vi "Launch Quad With Play and Pause.vi"   [LabVIEW 2017]
uses:
  ExampleSimpleRootModel/SimpleRootModel.lvclass
  C:/Git/mva-framework/gpm_packages/@cs/mva-core/Source/IObserver/IObserver/IObserver.lvclass
  C:/Git/mva-framework/gpm_packages/@cs/mva-core/Source/IModel/IModel/IModel.lvclass
  TwoPaneViewManager/TwoPaneViewManager.lvclass
  C:/Git/mva-framework/gpm_packages/@cs/mva-viewable/Source/IViewManager/IViewManager/IViewManager.lvclass
  C:/Git/mva-framework/gpm_packages/@cs/mva-viewable/Source/IViewable/IViewable/IViewable.lvclass
  SimpleViewModel/SimpleViewModel.lvclass
  C:/Git/mva-framework/gpm_packages/@cs/mva-viewable/Source/IViewModel/IViewModel/IViewModel.lvclass
  C:/Program Files (x86)/National Instruments/LabVIEW 2017/vi.lib/ActorFramework/Actor/Actor.lvclass
  gpm_packages/@cs/mva-core/Source/Mediator/Mediator/Mediator.lvclass
  C:/Git/mva-framework/gpm_packages/@cs/mva-core/Source/IMediator/IMediator/IMediator.lvclass
  <vilib>/ActorFramework/Message Enqueuer/Message Priority.ctl
  gpm_packages/@cs/mva-viewable/Source/IViewable/IViewable/View Position Enum.ctl
  SimpleChart/SimpleChart.lvclass
  VerticalSlide/VerticalSlide.lvclass
  PauseResumeButtons/PauseResumeButtons.lvclass
  gpm_packages/@cs/mva-viewable/Source/IViewManager/IViewManager Messages/Launch Nested Views Msg/Launch Nested Views Msg.lvclass/Launch Nested Views Msg.ctl
  gpm_packages/@cs/mva-viewable/Source/IViewManager/IViewManager/IViewManager.lvclass/IViewManager.ctl
  gpm_packages/@cs/event-logger/Source/Composed Log/LoggerReference/LoggerReference.lvclass/LoggerReference.ctl
  gpm_packages/@cs/mva-core/Source/IObserver/IObserver/IObserver.lvclass/IObserver.ctl
  gpm_packages/@cs/mva-core/Source/IMediator/IMediator/IMediator.lvclass/IMediator.ctl
  gpm_packages/@cs/mva-viewable/Source/IViewModel/IViewModel/IViewModel.lvclass/IViewModel.ctl
  gpm_packages/@cs/mva-viewable/Source/IViewable/IViewable Messages/Open Front Panel Msg/Open Front Panel Msg.lvclass/Open Front Panel Msg.ctl
  <vilib>/ActorFramework/Message Enqueuer/Message Enqueuer.lvclass/Message Enqueuer.ctl
  8aff559b-a38a-441b-bf19-c3bc83e17258.vi
  gpm_packages/@cs/mva-viewable/Source/IViewManager/IViewManager Messages/Launch Nested Views Msg/Pack Launch Nested Views Msg.vi
  8aff559b-a38a-441b-bf19-c3bc83e17258.vi/252d6523-7b57-4604-b517-1515f9ae2a9c.vi
  gpm_packages/@cs/mva-core/Source/IObserver/IObserver/Configure Observer Logging.vi
  gpm_packages/@cs/mva-viewable/Source/IViewModel/IViewModel/Write Startup Model-View Configuration.vi
  gpm_packages/@cs/mva-core/Source/IMediator/IMediator/Configure Mediator.vi
  <vilib>/ActorFramework/Message Enqueuer/Enqueue.vi
  gpm_packages/@cs/event-logger/Source/Composed Log/LoggerReference/Return Aggregate Queues.vi
  gpm_packages/@cs/event-logger/Source/Composed Log/LoggerReference/Add Aggregate Log.vi
  8aff559b-a38a-441b-bf19-c3bc83e17258.vi/252d6523-7b57-4604-b517-1515f9ae2a9c.vi/7a2ee304-0641-4048-9d5c-5dff84affc91.vi
  gpm_packages/@cs/mva-viewable/Source/IViewManager/IViewManager/Write Startup Launch Nested Views Msg.vi
  gpm_packages/@cs/event-logger/Source/Composed Log/LoggerReference/Send Add Sink.vi
  gpm_packages/@cs/event-logger/Source/Text File Sink/Text File Sink.lvclass
  C:/Git/mva-framework/gpm_packages/@cs/event-logger/Source/Composed Log/Log Sink/Log Sink.lvclass
  Source/ViewManager/QuadViewManager/QuadViewManager.lvclass
  gpm_packages/@cs/mva-viewable/Source/IViewModel/IViewModel/IViewModel.lvclass
  gpm_packages/@cs/mva-viewable/Source/IViewable/IViewable Messages/Open Front Panel Msg/Open Front Panel Msg.lvclass
  C:/Program Files (x86)/National Instruments/LabVIEW 2017/vi.lib/ActorFramework/Message/Message.lvclass
  gpm_packages/@cs/event-logger/Source/Composed Log/Application Logger/Launch Worker Loop.vi
  gpm_packages/@cs/event-logger/Source/Composed Log/LoggerReference/Initialize Logger Instance.vi
  <vilib>/ActorFramework/Message Priority Queue/Priority Enqueue.vi
  gpm_packages/@cs/mva-viewable/Source/IViewManager/IViewManager Messages/Launch Nested Views Msg/Launch Nested Views Msg.lvclass
  gpm_packages/@cs/event-logger/Source/Composed Log/LoggerReference/LoggerReference.lvclass
  gpm_packages/@cs/event-logger/Source/Composed Log/IErrorFormat/IErrorFormat.lvclass
  gpm_packages/@cs/event-logger/Source/Composed Log/Log Sink/Log Sink.lvclass
  gpm_packages/@cs/mva-viewable/Source/IViewable/IApplicationStyle/IApplicationStyle.lvclass
  <vilib>/ActorFramework/Actor/Actor.lvclass
  <vilib>/ActorFramework/Message Enqueuer/Message Enqueuer.lvclass
  gpm_packages/@cs/mva-viewable/Source/IViewable/IViewable/IViewable.lvclass
  gpm_packages/@cs/mva-viewable/Source/IViewManager/IViewManager/IViewManager.lvclass
panel:
  # "This example launches a QuadViewManager with other Viewables nested inside"
types:
  T1 = typedef "IViewable.lvlib/IViewable.lvclass/View Position Enum.ctl" = enum16{"Centered", "Maximized", "Minimized", "Custom", "Unchanged"}
  T2 = typedef "Actor Framework.lvlib/Message Enqueuer.lvclass/Message Priority.ctl" = enum16{"Low", "Normal", "High"}
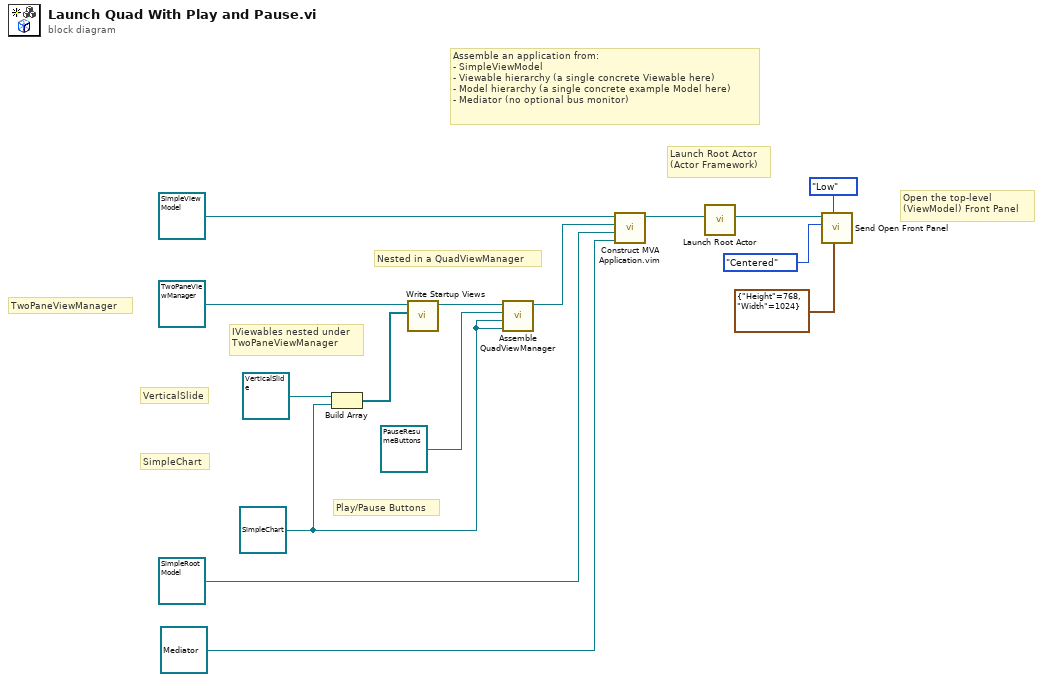
[diagram p0: block diagram]
diagram:
  w2 = refnum<class "SimpleChart.lvclass"> refnum ("MVAExamples.lvlib:SimpleChart.lvclass")
  # "Play/Pause Buttons"
  # "Nested in a QuadViewManager"
  # "SimpleChart"
  # "VerticalSlide"
  # "IViewables nested under \nTwoPaneViewManager"
  # "TwoPaneViewManager"
  # "Open the top-level\n(ViewModel) Front Panel"
  # "Launch Root Actor\n(Actor Framework)"
  # "Assemble an application from:\n- SimpleViewModel\n- Viewable hierarchy (a single concrete Viewable here)\n- Model hierarchy (a single concrete example Model here)\n- Mediator (no optional bus monitor)"
  n1 = Build Array(refnum<class "VerticalSlide.lvclass"> refnum ("MVAExamples.lvlib:VerticalSlide.lvclass"), w2) -> (w7:refnum<class "IViewable.lvclass">[])
  n2 = call "Write Startup Views.vi"("Startup Views"=w7, "IViewManager in"=refnum<class "TwoPaneViewManager.lvclass"> refnum ("MVAExamples.lvlib:TwoPaneViewManager.lvclass")) -> ("IViewManager out"=w3:refnum<class "TwoPaneViewManager.lvclass">)  [unwired: 9 in]
  n3 = call "Assemble QuadViewManager.vi"("Bottom-Right View"=w2, "Bottom-Left View"=w2, "Top-Right View"=refnum<class "PauseResumeButtons.lvclass"> refnum ("MVAExamples.lvlib:PauseResumeButtons.lvclass"), "Top-Left View"=w3) -> ("QuadViewManager out"=w6:refnum<class "QuadViewManager.lvclass">)  [unwired: 7 in]
  n4 = call "Construct MVA Application.vim"("Mediator Type"=refnum<class "Mediator.lvclass"> refnum ("Mediator.lvlib:Mediator.lvclass"), "Model Type"=refnum<class "SimpleRootModel.lvclass"> refnum ("MVAExamples.lvlib:SimpleRootModel.lvclass"), "Startup View Configuration"=w6, "IViewModel In"=refnum<class "SimpleViewModel.lvclass"> refnum ("MVAExamples.lvlib:SimpleViewModel.lvclass")) -> ("IViewModel Out"=w12:refnum<class "SimpleViewModel.lvclass">)  [unwired: 7 in]
  n5 = call <vilib>:"Launch Root Actor.vi"("Actor"=w12) -> ("Actor's Enqueuer"=w11:refnum<class "Message Enqueuer.lvclass">)  [unwired: 9 in, 1 out]
  n6 = call "Send Open Front Panel.vi"("Custom Window Size"=cluster{"Height":i16, "Width":i16} {"Height"=768, "Width"=1024}, "Message Priority (Normal)"=Message_Priority."Low", "Position"=View_Position_Enum."Centered", "Message Enqueuer"=w11) -> ()  [unwired: 6 in, 2 out]
